vi "svx_Configure Source (DAQmx).vi"(0 "acquisition task in":T3={"AI device settings"={"AI DAQmx TaskID"="", "response"=[]}, "acquisition type"=enum."Finite", "measurement settings"={"AI sampling frequency"=51200.0, "AO sampling frequency"=51200.0, "AI block size"=0, "AO block Size"=0, "block duration [ms]"=100.0, "number of AI channels"=0, "device propagation delay [samples]"=0.0, "DUT propagation time [s]"=0.0}, "settling settings"={"settle time"=0.015599999576807022, "settle cycles"=5}, "integration settings"={"integration time"=0.015599999576807022, "integration cycles"=5}, "AO device settings"={"AO DAQmx taskID"="", "excitation"=[]}, "acquisition accounting"={"initial read size [samples]"=0, "read offset [samples]"=0, "read length [samples]"=0, "blocks to settle [samples]"=0, "min delay until transition [samples]"=0}, "frequency range"={"start frequency"=0.015599999576807022, "stop frequency"=5.0}, "block type"=enum."Initialize", "source settings"={"signal type"=enum."Dual tone (IMD)", "frequency"=0.0, "total amplitude"=0.0, "frequencies"=[1.0], "relative amplitudes"=[1.0], "offset"=1.0, "total amplitude list"=[1.0], "ramping rate"=0.0}, "chirp settings"={"amplitude"=0.0, "frequency range"={"start (Hz)"=20.0, "stop (Hz)"=20000.0, "frequency spacing"=enum."Logarithmic"}, "sampling info"={"Fs"=50000.0, "chirp duration [s]"=3.0}, "initial states"={"frequency [Hz]"=20.0, "phase [rad]"=0.0, "elapsed time [s]"=0.0}, "frequency slope"=0.0, "maximum harmonic"=0, "prefix len [samples]"={"integer"=0, "fractional"=0.0}}} {"chirp settings"."frequency slope" format="%.2f"; "chirp settings"."prefix len [samples]"."fractional" format="%.2p"; "chirp settings"."initial states"."elapsed time [s]" format="%.2f"; "chirp settings"."initial states"."phase [rad]" format="%.2f"; "chirp settings"."initial states"."frequency [Hz]" format="%.2f"; "chirp settings"."sampling info"."chirp duration [s]" format="%.2f"; "chirp settings"."sampling info"."Fs" format="%.2p"; "chirp settings"."frequency range"."stop (Hz)" format="%.2f"; "chirp settings"."frequency range"."start (Hz)" format="%.2f"; "chirp settings"."amplitude" format="%.2f"; "source settings"."total amplitude" format="%.2f"; "source settings"."relative amplitudes" format="%.2f"; "source settings"."frequencies" format="%.2f"; "source settings"."total amplitude list" format="%.2f"; "source settings"."ramping rate" format="%.4f"; "source settings"."offset" format="%.2f"; "source settings"."frequency" format="%.2f"; "frequency range"."stop frequency" format="%.2f"; "frequency range"."start frequency" format="%.2f"; "AO device settings"."excitation"."AO channel settings"."terminal config" items=["Default"=-1, "Differential"=10106, "Pseudodifferential"=12529]; "AI device settings"."response"."AI channel settings"."DSA channel settings"."IEPE current [mA]" min=0.0 max=20.0 format="%.1f"; "AI device settings"."response"."AI channel settings"."DSA channel settings"."coupling" items=["AC"=10045, "DC"=10050, "GND"=10066]; "AI device settings"."response"."AI channel settings"."min value [V]" format="%.2f"; "AI device settings"."response"."AI channel settings"."terminal config" items=["Default"=-1, "RSE"=10083, "NRSE"=10078, "Differential"=10106, "Pseudodifferential"=12529]; "AI device settings"."response"."AI channel settings"."max value [V]" format="%.2f"; "integration settings"."integration time" format="%.2p"; "settling settings"."settle time" format="%.2p"; "measurement settings"."DUT propagation time [s]" format="%.2f"; "measurement settings"."AO sampling frequency" format="%.2f"; "measurement settings"."AI sampling frequency" format="%.2f"}, 1 "signal type":T2(ring), 2 "chirp settings":T1={"chirp duration [s]"=3.0, "frequency spacing"=enum."Logarithmic"}, 5 "sine frequency":dbl=1000.0 format="%.2f", 7 "total amplitude":dbl format="%.2f", 9 "amplitude-sweep amplitudes":dbl[](array[numeric]) format="%.2f", 11 "error in (no error)":errorcluster, 12 "IMD standard":T8(ring), 13 "custom IMD signal":T7={"IMD type"=enum."CCIF/Twin-Tone", "low-frequency tone"=14000.0, "high-frequency tone"=15000.0, "amplitude ratio"=1.0, "maximum order"=5} {"amplitude ratio" format="%.1f"; "high-frequency tone" format="%.2f"; "low-frequency tone" format="%.2f"}, 14 "multitone parameters":T9 {"component frequencies" format="%.2f"; "relative amplitudes" format="%.2f"}) -> (4 "acquisition task out":T3={"AI device settings"={"AI DAQmx TaskID"="", "response"=[]}, "acquisition type"=enum."Finite", "measurement settings"={"AI sampling frequency"=51200.0, "AO sampling frequency"=51200.0, "AI block size"=0, "AO block Size"=0, "block duration [ms]"=100.0, "number of AI channels"=0, "device propagation delay [samples]"=0.0, "DUT propagation time [s]"=0.0}, "settling settings"={"settle time"=0.015599999576807022, "settle cycles"=5}, "integration settings"={"integration time"=0.015599999576807022, "integration cycles"=5}, "AO device settings"={"AO DAQmx taskID"="", "excitation"=[]}, "acquisition accounting"={"initial read size [samples]"=0, "read offset [samples]"=0, "read length [samples]"=0, "blocks to settle [samples]"=0, "min delay until transition [samples]"=0}, "frequency range"={"start frequency"=0.015599999576807022, "stop frequency"=5.0}, "block type"=enum."Initialize", "source settings"={"signal type"=enum."Dual tone (IMD)", "frequency"=0.0, "total amplitude"=0.0, "frequencies"=[1.0], "relative amplitudes"=[1.0], "offset"=1.0, "total amplitude list"=[1.0], "ramping rate"=0.0}, "chirp settings"={"amplitude"=0.0, "frequency range"={"start (Hz)"=20.0, "stop (Hz)"=20000.0, "frequency spacing"=enum."Logarithmic"}, "sampling info"={"Fs"=50000.0, "chirp duration [s]"=3.0}, "initial states"={"frequency [Hz]"=20.0, "phase [rad]"=0.0, "elapsed time [s]"=0.0}, "frequency slope"=0.0, "maximum harmonic"=0, "prefix len [samples]"={"integer"=0, "fractional"=0.0}}} {"chirp settings"."frequency slope" format="%.2f"; "chirp settings"."prefix len [samples]"."fractional" format="%.2p"; "chirp settings"."initial states"."elapsed time [s]" format="%.2f"; "chirp settings"."initial states"."phase [rad]" format="%.2f"; "chirp settings"."initial states"."frequency [Hz]" format="%.2f"; "chirp settings"."sampling info"."chirp duration [s]" format="%.2f"; "chirp settings"."sampling info"."Fs" format="%.2p"; "chirp settings"."frequency range"."stop (Hz)" format="%.2f"; "chirp settings"."frequency range"."start (Hz)" format="%.2f"; "chirp settings"."amplitude" format="%.2f"; "source settings"."total amplitude" format="%.2f"; "source settings"."relative amplitudes" format="%.2f"; "source settings"."frequencies" format="%.2f"; "source settings"."total amplitude list" format="%.2f"; "source settings"."ramping rate" format="%.4f"; "source settings"."offset" format="%.2f"; "source settings"."frequency" format="%.2f"; "frequency range"."stop frequency" format="%.2f"; "frequency range"."start frequency" format="%.2f"; "AO device settings"."excitation"."AO channel settings"."terminal config" items=["Default"=-1, "Differential"=10106, "Pseudodifferential"=12529]; "AI device settings"."response"."AI channel settings"."DSA channel settings"."IEPE current [mA]" min=0.0 max=20.0 format="%.1f"; "AI device settings"."response"."AI channel settings"."DSA channel settings"."coupling" items=["AC"=10045, "DC"=10050, "GND"=10066]; "AI device settings"."response"."AI channel settings"."min value [V]" format="%.2f"; "AI device settings"."response"."AI channel settings"."terminal config" items=["Default"=-1, "RSE"=10083, "NRSE"=10078, "Differential"=10106, "Pseudodifferential"=12529]; "AI device settings"."response"."AI channel settings"."max value [V]" format="%.2f"; "integration settings"."integration time" format="%.2p"; "settling settings"."settle time" format="%.2p"; "measurement settings"."DUT propagation time [s]" format="%.2f"; "measurement settings"."AO sampling frequency" format="%.2f"; "measurement settings"."AI sampling frequency" format="%.2f"}, 15 "error out":errorcluster)   [LabVIEW 2017]
doc: "This example VI allows you to configure the source that will be used for the synchronized AO/AI measurment.\n\nSet <B>signal type</B> to specify the nature of the excitation signal (e.g. whether the test signal is a sinewave, a multitone, a chirp, or noise).\n\nSet <B>total amplitude</B> to set the maximum amplitude of the time-domain excitation signal.\n\nOnly the source parameters associated with the selected signal type are configured."
uses:
  <vilib>/addons/Sound and Vibration/Example Support/Audio/DAQmx/svx_Acquisition Task (DAQmx).ctl
  <vilib>/addons/_NISVFA/_Shared subVIs/Controls/svc_Channel Settings.ctl
  <vilib>/addons/_NISVFA/_Shared subVIs/Controls/svc_DSA Channel Settings.ctl
  <vilib>/addons/_NISVFA/_Generation/subVIs/sv_Chirp Settings.ctl
  <vilib>/addons/_NISVFA/_Generation/SoundVib_Generation.lvlib
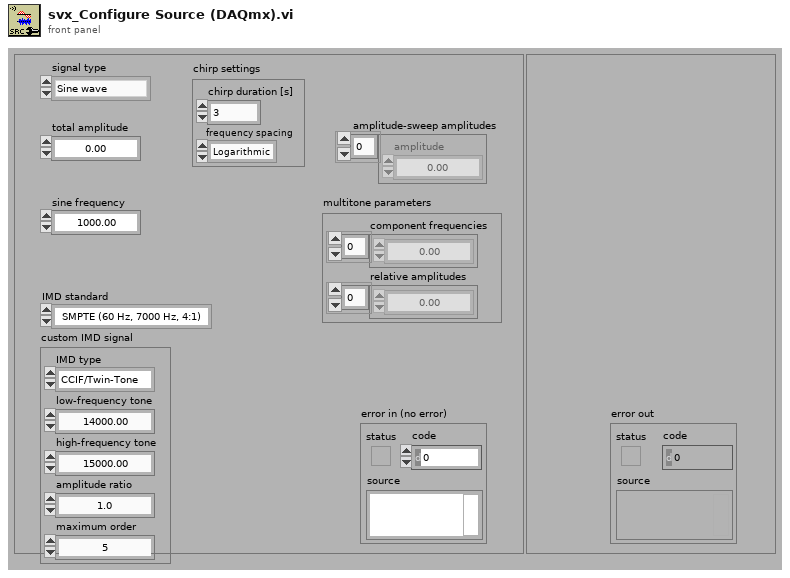
[diagram p1: front panel]
types:
  T1 = cluster{"chirp duration [s]":dbl, "frequency spacing":enum16{"Linear", "Logarithmic"}}
  T2 = enum16{"Sine wave", "Dual tone (IMD)", "Multitone", "Chirp", "Frequency flat chirp", "Uniform white noise", "Gaussian white noise", "Pink noise", "PRN"}
  T3 = typedef "svx_Acquisition Task (DAQmx).ctl" = cluster{"AI device settings":cluster{"AI DAQmx TaskID":refnum<k21>, "response":cluster{"AI physical channel":tag, "AI channel settings":T4}[]}, "acquisition type":enum16{"Finite", "Averaged", "Settled", "Amplitude Sweep", "Stepped Frequency Sweep", "Continuous Frequency Sweep"}, "measurement settings":cluster{"AI sampling frequency":dbl, "AO sampling frequency":dbl, "AI block size":i32, "AO block Size":i32, "block duration [ms]":dbl, "number of AI channels":i32, "device propagation delay [samples]":dbl, "DUT propagation time [s]":dbl}, "settling settings":cluster{"settle time":dbl, "settle cycles":i32}, "integration settings":cluster{"integration time":dbl, "integration cycles":i32}, "AO device settings":cluster{"AO DAQmx taskID":refnum<k21>, "excitation":cluster{"AO physical channel":tag, "AO channel settings":cluster{"maximum value (10 V)":dbl, "minimum value (10 V)":dbl, "terminal config":i32}}[]}, "acquisition accounting":cluster{"initial read size [samples]":i32, "read offset [samples]":i32, "read length [samples]":i32, "blocks to settle [samples]":i32, "min delay until transition [samples]":i32}, "frequency range":cluster{"start frequency":dbl, "stop frequency":dbl}, "block type":enum16{"Initialize", "Settle", "Integrate"}, "source settings":cluster{"signal type":enum16{"Sine wave", "Dual tone (IMD)", "Multitone", "Chirp", "Frequency flat chirp", "Uniform white noise", "Gaussian white noise", "Pink noise", "PRN", "Continuous swept-sine"}, "frequency":dbl, "total amplitude":dbl, "frequencies":dbl[], "relative amplitudes":dbl[], "offset":dbl, "total amplitude list":dbl[], "ramping rate":dbl}, "chirp settings":T6}
  T4 = typedef "svc_Channel Settings.ctl" = cluster{"max value [V]":dbl, "min value [V]":dbl, "terminal config":i32, "DSA channel settings":T5}
  T5 = typedef "svc_DSA Channel Settings.ctl" = cluster{"coupling":i32, "enable IEPE excitation":bool, "IEPE current [mA]":dbl}
  T6 = typedef "SoundVib_Generation.lvlib/sv_Chirp Settings.ctl" = cluster{"amplitude":dbl, "frequency range":cluster{"start (Hz)":dbl, "stop (Hz)":dbl, "frequency spacing":enum16{"Linear", "Logarithmic"}}, "sampling info":cluster{"Fs":dbl, "chirp duration [s]":dbl}, "initial states":cluster{"frequency [Hz]":dbl, "phase [rad]":dbl, "elapsed time [s]":dbl}, "frequency slope":dbl, "maximum harmonic":i32, "prefix len [samples]":cluster{"integer":u32, "fractional":dbl}}
  T7 = cluster{"IMD type":enum16{"SMPTE/DIN", "CCIF/Twin-Tone"}, "low-frequency tone":dbl, "high-frequency tone":dbl, "amplitude ratio":dbl, "maximum order":i32}
  T8 = enum16{"SMPTE (60 Hz, 7000 Hz, 4:1)", "DIN (250 Hz, 8000 Hz, 4:1)", "CCIF (11 kHz, 12 kHz, 1:1)", "CCIF (19 kHz, 20 kHz, 1:1)", "Custom"}
  T9 = cluster{"component frequencies":dbl[], "relative amplitudes":dbl[]}
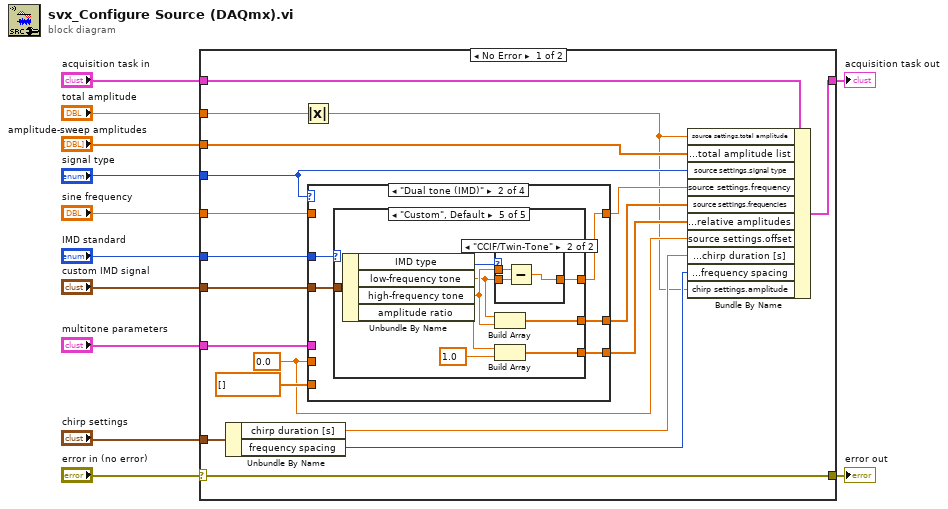
[diagram p0: block diagram]
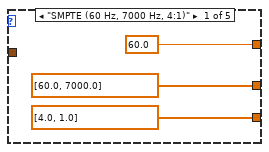
[diagram p3: hidden frame]
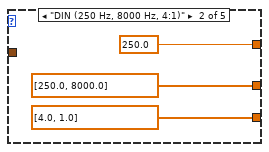
[diagram p4: hidden frame]
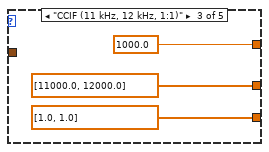
[diagram p5: hidden frame]
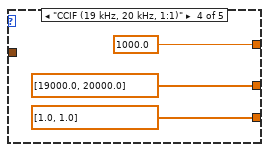
[diagram p6: hidden frame]
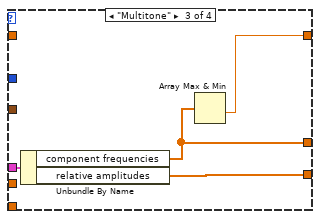
[diagram p8: hidden frame]
diagram:
  n1 = case shown="No Error" "error in (no error)" {
    selector: "error in (no error)" -> [w30 w71]
    tunnel: [w31 w70] -> w12
    tunnel: "acquisition task in" -> [w20 w70]
    tunnel: "signal type" -> [w15 _]
    tunnel: [w30 w71] -> w9
    tunnel: "amplitude-sweep amplitudes" -> [w21 _]
    tunnel: "custom IMD signal" -> [w28 _]
    tunnel: "multitone parameters" -> [w27 _]
    tunnel: "IMD standard" -> [w29 _]
    tunnel: "total amplitude" -> [w14 _]
    tunnel: "sine frequency" -> [w19 _]
    tunnel: "chirp settings" -> [w18 _]
    frame No Error {
      w24 = 0.0 ("amplitude")
      n2 = Unbundle By Name(w18) -> ("chirp duration [s]"=w17:dbl, "frequency spacing"=w16:enum16{"Linear", "Logarithmic"})
      n3 = Absolute Value(x=w14) -> (abs(x)=w13:dbl)
      n4 = case shown="\"Dual tone (IMD)\"" w15 {
        tunnel: w28 -> [_ w37 _ _]
        tunnel: w27 -> [_ _ w67 _]
        tunnel: [w32 w34 w64 w69] -> w26
        tunnel: w24 -> [_ _ _ w69]
        tunnel: dbl[] [] ("source settings.frequencies") -> [w33 _ _ w68]
        tunnel: [w33 w35 w66 w68] -> w23
        tunnel: [w33 w36 w65 w68] -> w22
        tunnel: w29 -> [_ w38 _ _]
        tunnel: w19 -> [w32 _ _ _]
        frame "Sine wave", Default {
        }
        frame "Dual tone (IMD)" {
          n5 = case shown="\"Custom\", Default" w38 {
            tunnel: w37 -> [_ _ _ _ w59]
            tunnel: [dbl[] [60.0, 7000.0] ("source settings.frequencies") dbl[] [250.0, 8000.0] ("source settings.frequencies") dbl[] [11000.0, 12000.0] ("source settings.frequencies") dbl[] [19000.0, 20000.0] ("source settings.frequencies") w58] -> w36
            tunnel: [dbl[] [4.0, 1.0] ("source settings.frequencies") dbl[] [4.0, 1.0] ("source settings.frequencies") dbl[] [1.0, 1.0] ("source settings.frequencies") dbl[] [1.0, 1.0] ("source settings.frequencies") w57] -> w35
            tunnel: [60.0 ("low-frequency tone") 250.0 ("low-frequency tone") 1000.0 ("low-frequency tone") 1000.0 ("low-frequency tone") w51] -> w34
            frame "SMPTE (60 Hz, 7000 Hz, 4:1)" {
            }
            frame "DIN (250 Hz, 8000 Hz, 4:1)" {
            }
            frame "CCIF (11 kHz, 12 kHz, 1:1)" {
            }
            frame "CCIF (19 kHz, 20 kHz, 1:1)" {
            }
            frame "Custom", Default {
              n6 = Unbundle By Name(w59) -> ("IMD type"=w55:enum16{"SMPTE/DIN", "CCIF/Twin-Tone"}, "low-frequency tone"=w52:dbl, "high-frequency tone"=w53:dbl, "amplitude ratio"=w54:dbl)
              n7 = case shown="\"CCIF/Twin-Tone\"" w55 {
                tunnel: w53 -> [_ w63]
                tunnel: w52 -> [w60 w62]
                tunnel: [w60 w61] -> w51
                frame "SMPTE/DIN", Default {
                }
                frame "CCIF/Twin-Tone" {
                  n8 = Subtract(x=w63, y=w62) -> (x-y=w61:dbl)
                }
              }
              n9 = Build Array(w52, w53) -> (w58:dbl[])
              n10 = Build Array(w54, 1.0 ("element")) -> (w57:dbl[])
            }
          }
        }
        frame "Multitone" {
          n11 = Unbundle By Name(w67) -> ("component frequencies"=w65:dbl[], "relative amplitudes"=w66:dbl[])
          n12 = Array Max & Min(array=w65) -> (min value=w64:dbl)  [unwired: 3 out]
        }
        frame "Chirp".."PRN" {
        }
      }
      n13 = Bundle By Name(cluster=w20, "source settings.total amplitude"=w13, "source settings.total amplitude list"=w21, "source settings.signal type"=w15, "source settings.frequency"=w26, "source settings.frequencies"=w22, "source settings.relative amplitudes"=w23, "source settings.offset"=w24, "chirp settings.sampling info.chirp duration [s]"=w17, "chirp settings.frequency range.frequency spacing"=w16, "chirp settings.amplitude"=w13) -> (w31:T3)
    }
    frame Error {
    }
  }
  "acquisition task out" <- w12
  "error out" <- w9
